vi "Jacobian Setup.vi"(2 "error in (no error)":errorcluster, 3 "LBCB Selected":T1) -> (0 "error out":errorcluster)   [LabVIEW 2009]
uses:
  lib/Data Access Objects/Metadata/LBCB Number.ctl
  lib/Data Access Objects/Metadata/Persistant DAO Actions.ctl
  Update Actions.ctl
panel:
  in  "L2 Default Stiffness Jacobian":dbl[][](array[numeric])=[[100000000.0, 0.0, 0.0, 0.0, 0.0, 0.0], [0.0, 100000000.0, 0.0, 0.0, 0.0, 0.0], [0.0, 0.0, 100000000.0, 0.0, 0.0, 0.0], [0.0, 0.0, 0.0, 100000000.0, 0.0, 0.0], [0.0, 0.0, 0.0, 0.0, 100000000.0, 0.0], [0.0, 0.0, 0.0, 0.0, 0.0, 100000000.0]]
  in  "L1 Default Stiffness Jacobian":dbl[][](array[numeric])=[[100000000.0, 0.0, 0.0, 0.0, 0.0, 0.0], [0.0, 100000000.0, 0.0, 0.0, 0.0, 0.0], [0.0, 0.0, 100000000.0, 0.0, 0.0, 0.0], [0.0, 0.0, 0.0, 100000000.0, 0.0, 0.0], [0.0, 0.0, 0.0, 0.0, 100000000.0, 0.0], [0.0, 0.0, 0.0, 0.0, 0.0, 100000000.0]]
  in  "Cancel":bool
  in  "OK":bool
  in  "Stiffness Jacobian":dbl[][](array[numeric])=[[100000000.0, 0.0, 0.0, 0.0, 0.0, 0.0], [0.0, 100000000.0, 0.0, 0.0, 0.0, 0.0], [0.0, 0.0, 100000000.0, 0.0, 0.0, 0.0], [0.0, 0.0, 0.0, 100000000.0, 0.0, 0.0], [0.0, 0.0, 0.0, 0.0, 100000000.0, 0.0], [0.0, 0.0, 0.0, 0.0, 0.0, 100000000.0]]
  # "dx (in)"
  # "dy (in)"
  # "dz (in)"
  # "dRx (rad)"
  # "dRy (rad)"
  # "dRz (rad)"
  # "dFx (lb) ="
  # "dFy (lb) ="
  # "dFz (lb)  ="
  # "dMx (lb*in)  ="
  # "dMy (lb*in)  ="
  # "dMz (lb*in)  ="
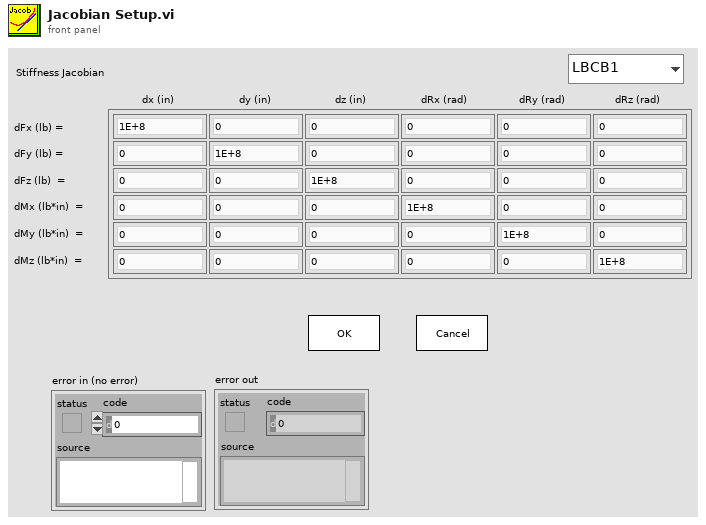
[diagram p1: front panel]
types:
  T1 = typedef "LBCB Number.ctl" = enum16{"LBCB1", "LBCB2"}
  T2 = typedef "Update Actions.ctl" = enum16{"Update", "Exit"}
  T3 = typedef "Persistant DAO Actions.ctl" = enum16{"Init", "Get", "Set", "Load", "Save"}
  T4 = typedef "Stiffness Matrix.ctl" = dbl[][]
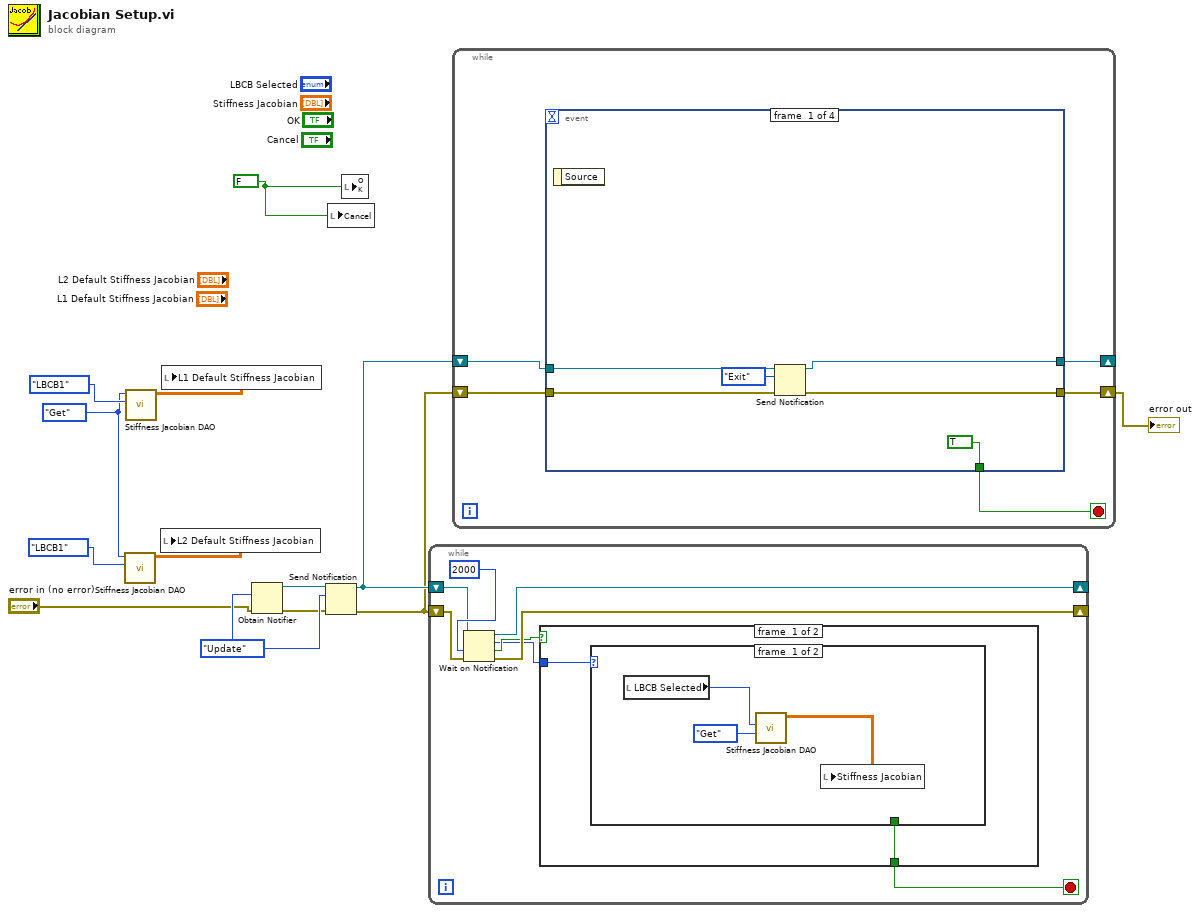
[diagram p0: block diagram]
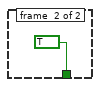
[diagram p2: hidden frame]
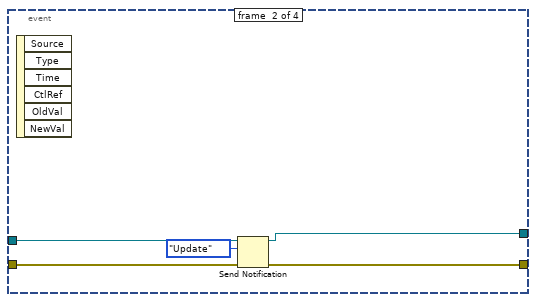
[diagram p4: hidden frame]
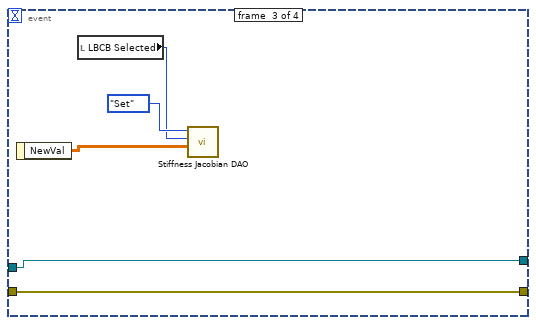
[diagram p5: hidden frame]
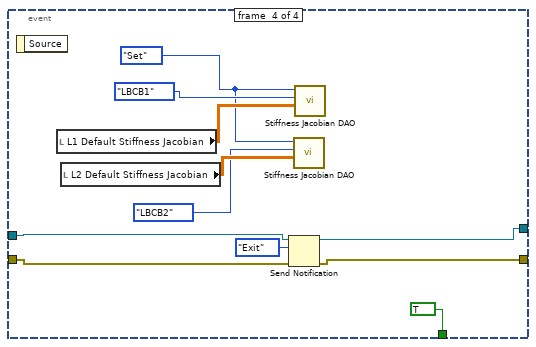
[diagram p6: hidden frame]
diagram:
  w1 = FALSE ("OK")
  w8 = Update_Actions."Update" ("Update Actions")
  w9 = Persistant_DAO_Actions."Get" ("Stiffness Jacobian Datastore Actions")
  n1 = call "Stiffness Jacobian DAO.vi"("LBCB Number"=LBCB_Number."LBCB1", "Actions"=w9) -> ("Stiffness Jacobian Out"=w11:T4)  [unwired: 3 in, 6 out]
  n2 = call "Stiffness Jacobian DAO.vi"("LBCB Number"=LBCB_Number."LBCB1", "Actions"=w9) -> ("Stiffness Jacobian Out"=w13:T4)  [unwired: 3 in, 6 out]
  n3 = local write "L2 Default Stiffness Jacobian"(w11) -> ()
  n4 = local write "L1 Default Stiffness Jacobian"(w13) -> ()
  n5 = Obtain Notifier(notification data type=w8, error in (no error)="error in (no error)") -> (notifier out=w7:refnum<notifier>, error out=w6:errorcluster)  [unwired: 1 in, 2 out]
  n6 = Send Notification(notification=w8, notifier=w7, error in (no error)=w6) -> (notifier out=w5:refnum<notifier>, error out=w3:errorcluster)
  n7 = local write "Cancel"(w1) -> ()
  n8 = local write "OK"(w1) -> ()
  n9 = while {
    shift-right: [w17] -> _
    shift-left: w5 -> [w19]
    shift-right: [w18] -> _
    shift-left: w3 -> [w20]
    stop <- w14 stop-if-true
    n10 = Wait on Notification(notifier=w19, timeout in ms (-1)=2000, error in (no error)=w20) -> (notifier out=w17:refnum<notifier>, notification=w15:T2, timed out?=w16:bool, error out=w18:errorcluster)  [unwired: 1 out]
    n11 = case shown="False" w16 {
      tunnel: w15 -> [w23 _]
      tunnel: [w22 _] -> w14
      frame #0 {
        n12 = case shown="\"Update\"" w23 {
          tunnel: [_ TRUE] -> w22
          frame #0 {
            n13 = local read "LBCB Selected"() -> (w24:T1)
            n14 = call "Stiffness Jacobian DAO.vi"("LBCB Number"=w24, "Actions"=Persistant_DAO_Actions."Get" ("Stiffness Jacobian Datastore Actions")) -> ("Stiffness Jacobian Out"=w25:T4)  [unwired: 3 in, 6 out]
            n15 = local write "Stiffness Jacobian"(w25) -> ()
          }
          frame #1 {
          }
        }
      }
      frame #1 {
      }
    }
  }
  n16 = while {
    shift-right: [w29] -> _
    shift-left: w5 -> [w31]
    shift-right: [w28] -> w2
    shift-left: w3 -> [w30]
    stop <- w32 stop-if-true
    n17 = event shown="[1] \"LBCB Selected\": Value Change" {
      selector: _ -> [_ _ _ _]
      dyn-events: _ -> [_ _ _ _]
      timeout: _ -> [_ _ _ _]
      tunnel: [TRUE _ _ TRUE] -> w32
      tunnel: w31 -> [w37 w43 w45 w52]
      tunnel: w30 -> [w36 w42 w44 w50]
      tunnel: [w34 w40 w45 w51] -> w29
      tunnel: [w33 w39 w44 w49] -> w28
      event #0 {
        n18 = event-data() -> ()  [unwired: 2 out]
        n19 = Send Notification(notification=Update_Actions."Exit", notifier=w37, error in (no error)=w36) -> (notifier out=w34:refnum<notifier>, error out=w33:errorcluster)
      }
      event #1 {
        n20 = event-data() -> ()  [unwired: 7 out]
        n21 = Send Notification(notification=Update_Actions."Update", notifier=w43, error in (no error)=w42) -> (notifier out=w40:refnum<notifier>, error out=w39:errorcluster)
      }
      event #2 {
        n22 = event-data() -> ("NewVal"=w47:dbl[][])  [unwired: 1 out]
        n23 = local read "LBCB Selected"() -> (w46:T1)
        n24 = call "Stiffness Jacobian DAO.vi"("Stiffness Jacobian In"=w47, "LBCB Number"=w46, "Actions"=Persistant_DAO_Actions."Set" ("Stiffness Jacobian Datastore Actions")) -> ()  [unwired: 2 in, 7 out]
      }
      event #3 {
        w55 = Persistant_DAO_Actions."Set" ("Actions")
        n25 = event-data() -> ()  [unwired: 2 out]
        n26 = local read "L1 Default Stiffness Jacobian"() -> (w58:dbl[][])
        n27 = local read "L2 Default Stiffness Jacobian"() -> (w57:dbl[][])
        n28 = Send Notification(notification=Update_Actions."Exit", notifier=w52, error in (no error)=w50) -> (notifier out=w51:refnum<notifier>, error out=w49:errorcluster)
        n29 = call "Stiffness Jacobian DAO.vi"("Stiffness Jacobian In"=w57, "LBCB Number"=LBCB_Number."LBCB2", "Actions"=w55) -> ()  [unwired: 2 in, 7 out]
        n30 = call "Stiffness Jacobian DAO.vi"("Stiffness Jacobian In"=w58, "LBCB Number"=LBCB_Number."LBCB1", "Actions"=w55) -> ()  [unwired: 2 in, 7 out]
      }
    }
  }
  "error out" <- w2
